vi "remove_empty_group.vi"(10 "Group":string[](array[string]), 11 "TreeControl In":refnum<vi>) -> (3 "TreeControl Out":refnum<vi>)   [LabVIEW 2018]
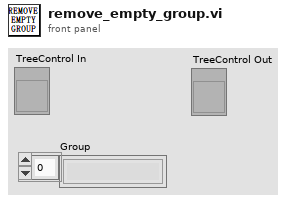
[diagram p1: front panel]
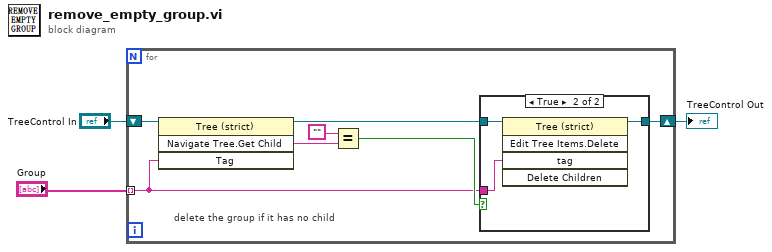
[diagram p0: block diagram]
diagram:
  n1 = for {
    shift-right: [w5] -> w2
    shift-left: "TreeControl In" -> [w8]
    tunnel: "Group" -> [w4] mode=indexing
    # "delete the group if it has no child"
    n2 = invoke class="Tree (strict)" method="Navigate Tree.Get Child"(reference=w8, "Tag"=w4) -> (reference out=w6:refnum<vi>, "Navigate Tree:Get Child"=w10:string)  [unwired: 2 in, 2 out]
    n3 = Equal?(x="", y=w10) -> (x = y?=w7:bool)
    n4 = case shown="True" w7 {
      tunnel: w6 -> [w11 w14]
      tunnel: [w11 w13] -> w5
      tunnel: w4 -> [_ w12]
      frame False {
      }
      frame True {
        n5 = invoke class="Tree (strict)" method="Edit Tree Items.Delete"(reference=w14, "tag"=w12) -> (reference out=w13:refnum<vi>)  [unwired: 3 in, 4 out]
      }
    }
  }
  "TreeControl Out" <- w2
